vi "Configuration 1.1 JSON Flatten.vi"(8 "error in (no error)":errorcluster, 11 "framework configuration 1.1":T2={"plugins"=[{"name"="Plugin", "components"=[], "cycle timing"={"priority"=10000, "decimation"=1, "offset"=0}, "threads"=[], "transfer groups"=[{"name"="Group", "direction"=0, "cycle timing"={"priority"=100, "decimation"=1, "offset"=0}, "thread index"=-1, "settings"=[], "transfers"=[{"name"="Transfer", "byte order"=0, "settings"=[], "channels"=[{"string offset"=0, "string data type"=2, "engine data type"=2, "name"="Channel", "settings"=[], "units"="V"}]}], "timeout behavior"=0}], "settings"=[]}]}) -> (0 "error out":errorcluster, 2 "dsf version":T1, 3 "dsf configuration json":string)   [LabVIEW 2019, in "DSF Core.lvlib" / "Configuration Session.lvclass"]
uses:
  Configuration Session.lvclass
  Typedefs/DSF Version Info.ctl
  DSF Core.lvlib
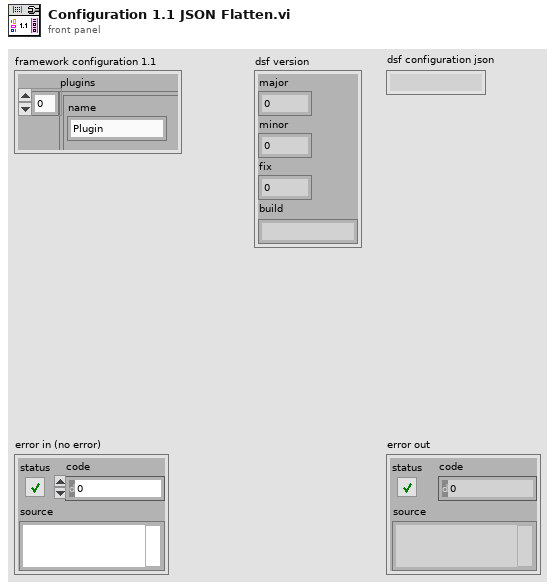
[diagram p1: front panel]
types:
  T1 = typedef "DSF Core.lvlib/DSF Version Info.ctl" = cluster{"major":u32, "minor":u32, "fix":u32, "build":string}
  T2 = cluster{"plugins":cluster{"name":string, "components":string[], "cycle timing":cluster{"priority":u64, "decimation":u64, "offset":u64}, "threads":cluster{"buffer converter settings":cluster{"key":string, "value":string}[], "transceiver settings":cluster{"key":string, "value":string}[], "custom settings":cluster{"key":string, "value":string}[], "processor":i32, "priority offset":i16}[], "transfer groups":cluster{"name":string, "direction":u8, "cycle timing":cluster{"priority":u64, "decimation":u64, "offset":u64}, "thread index":i32, "settings":cluster{"key":string, "value":string}[], "transfers":cluster{"name":string, "byte order":u8, "settings":cluster{"key":string, "value":string}[], "channels":cluster{"string offset":u64, "string data type":u8, "engine data type":u8, "name":string, "settings":cluster{"key":string, "value":string}[], "units":string}[]}[], "timeout behavior":u8}[], "settings":cluster{"key":string, "value":string}[]}[]}
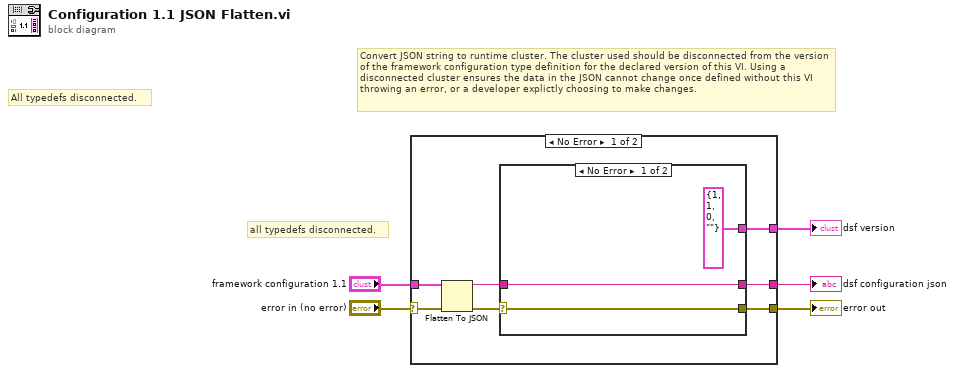
[diagram p0: block diagram]
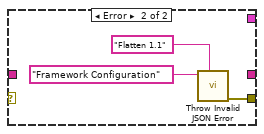
[diagram p2: hidden frame]
diagram:
  # "all typedefs disconnected."
  # "All typedefs disconnected."
  # "Convert JSON string to runtime cluster. The cluster used should be disconnected from the version of the framework configuration type definition for the declared version of this VI. Using a disconnected cluster ensures the data in the JSON cannot change once defined without this VI throwing an error, or a developer explictly choosing to make changes."
  n1 = case shown="No Error" "error in (no error)" {
    selector: "error in (no error)" -> [w9 w19]
    tunnel: [w11 w19] -> w5
    tunnel: "framework configuration 1.1" -> [w8 _]
    tunnel: [w7 _] -> w2
    tunnel: [w6 _] -> w1
    frame No Error {
      n2 = Flatten To JSON(anything=w8, error in (no error)=w9) -> (JSON string=w10:string, 11:w12:errorcluster)  [unwired: 1 in]
      n3 = case shown="No Error" w12 {
        selector: w12 -> [w15 _]
        tunnel: [w15 w18] -> w11
        tunnel: w10 -> [w14 _]
        tunnel: [w14 _] -> w7
        tunnel: [T1 {"major"=1, "minor"=1, "fix"=0, "build"=""} ("json version") _] -> w6
        frame No Error {
        }
        frame Error {
          n4 = call "Throw Invalid JSON Error.vi"("error source vi name"="Flatten 1.1", "name"="Framework Configuration") -> ("error out"=w18:errorcluster)  [unwired: 9 in]
        }
      }
    }
    frame Error {
    }
  }
  "dsf configuration json" <- w2
  "error out" <- w5
  "dsf version" <- w1
